vi "Test_Max_of_3.vi"() -> ()   [LabVIEW 2022 SP3]
panel:
  out "Numeric out":dbl
  in  "input 2":dbl
  in  "input 3":dbl
  in  "input 1":dbl
  in  "stop":bool
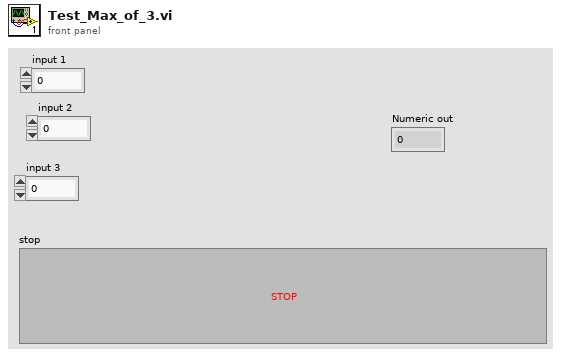
[diagram p1: front panel]
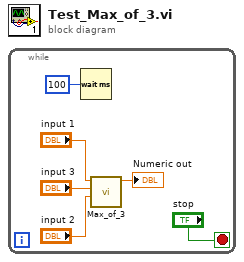
[diagram p0: block diagram]
diagram:
  n1 = while {
    stop <- "stop" stop-if-true
    n2 = Wait (ms)(milliseconds to wait=u32 100) -> ()  [unwired: 1 out]
    n3 = call "Max_of_3.vi"("input 2"="input 2", "input 3"="input 3", "input 1"="input 1") -> ("Numeric out"=→"Numeric out":dbl)  [unwired: 7 in, 1 out]
  }
